vi "LVDimInterface.dim_set_DNS_node.vi"(1 "DNS node":string, 5 "error in (no error)":errorcluster) -> (14 "success":i32, 19 "error out":errorcluster)   [LabVIEW 2014, in "LVDimInterface.lvlib"]
doc: "This routine can be called by a server or a client program before publishing or subscribing to any services in order to programmatically declare the node where the DNS is running. If this call is not used the environment variable DIM_DNS_NODE will be used instead.\n\nA list of node names separated by commas can be given as a parameter, in which case the server or the client will use the first name server found running from the list.\n\n\n\nHistory: 29-JUN-2006, Dietrich Beck\n\nCopyright (C)\nGesellschaft für Schwerionenforschung, GSI\nPlanckstr. 1\n64291 Darmstadt\nGermany\n\nContact: D.Beck@gsi.de \n\nThis program is free software; you can redistribute it and/or modify it under the terms of the \nGNU General Public License as published by the Free Software Foundation; either version 2 of the license, or (at your option) any later version.\n\nThis program is distributed in the hope that it will be useful, but WITHOUT ANY WARRANTY; without even the implied warranty of MERCHANTABILITY or FITNESS FOR A PARTICULAR PURPOSE. See the GNU General License for more details (http://www.gnu.org).\n\nGesellschaft für Schwerionenforschung, GSI\nPlanckstr. 1, 64291 Darmstadt, Germany\nFor all questions and ideas contact D. Beck.\nLast update: 16-DEC-2005"
uses:
  LVDimInterface.lvlib
  bin/libDimWrapper.dll
  bin/libDimWrapper.so
  bin/libDimWrapperSPL.dll
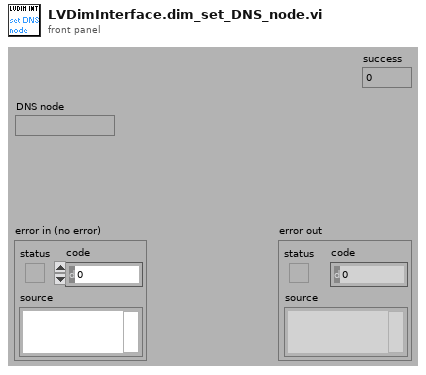
[diagram p1: front panel]
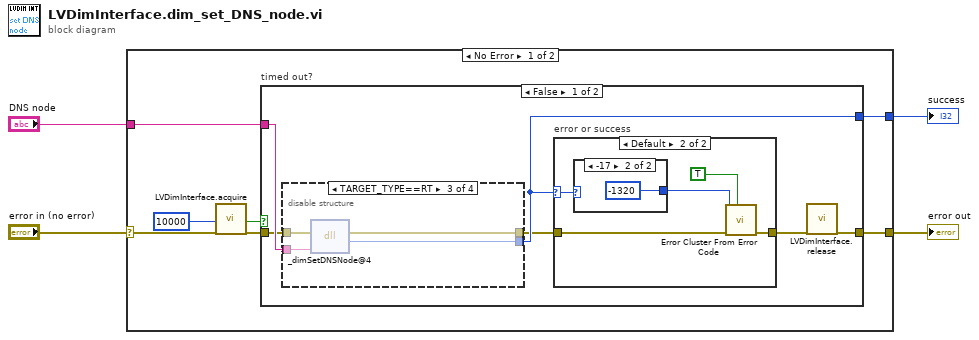
[diagram p0: block diagram]
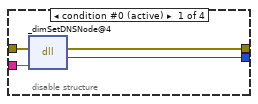
[diagram p2: hidden frame]
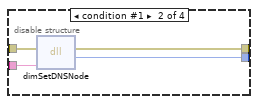
[diagram p3: hidden frame]
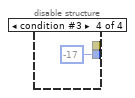
[diagram p4: hidden frame]
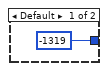
[diagram p6: hidden frame]
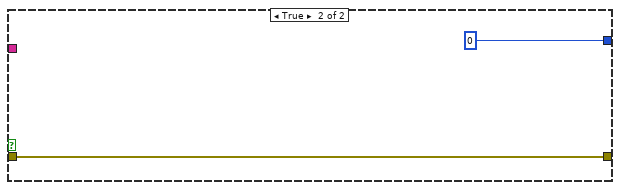
[diagram p7: hidden frame]
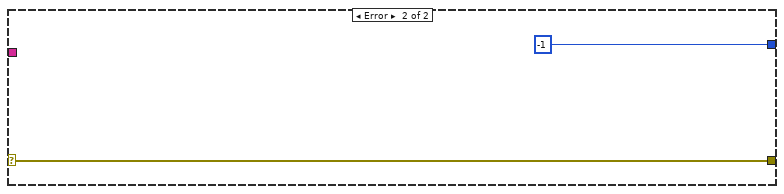
[diagram p8: hidden frame]
diagram:
  n1 = case shown="No Error" "error in (no error)" {
    selector: "error in (no error)" -> [w5 w42]
    tunnel: "DNS node" -> [w11 _]
    tunnel: [w10 -1 ("success")] -> w3
    tunnel: [w9 w42] -> w2
    frame No Error {
      n2 = call "LVDimInterface.acquire.vi"("ms timeout (10000)"=10000 ("ms timeout (-1)"), "error in (no error)"=w5) -> ("timed out"=w7:bool, "error out"=w8:errorcluster)  [unwired: 16 in]
      n3 = case "timed out?" shown="False" w7 {
        tunnel: w11 -> [w17 _]
        tunnel: [w16 0 ("success")] -> w10
        tunnel: [w12 w39] -> w9
        tunnel: w8 -> [w14 w39]
        frame False {
          n4 = disable-structure "Conditional Disable Structure" shown="TARGET_TYPE==RT" {
            disable-tunnel: w17 -> [w21 w25 w29 _]
            disable-tunnel: [w20 w24 w28 -17 ("success")] -> w16
            disable-tunnel: w14 -> [w19 w23 w27 _]
            disable-tunnel: [w18 w22 w26 _] -> w15
            frame condition #0 (active) {
              n5 = dll-call lib="D:/Git/CS-framework/CSlibraries/DimLVEvent/bin/libDimWrapper.dll" fn="_dimSetDNSNode@4" label="dimSetDNSNode"(error in=w19, "DNSNode"=w21) -> (error out=w18:errorcluster, "success"=w20:i32)  [unwired: 3 in, 1 out]
            }
            frame condition #1 {
              n6 = dll-call lib="D:/Git/CS-framework/CSlibraries/DimLVEvent/bin/libDimWrapper.so" fn="dimSetDNSNode"(error in=w23, "DNSNode"=w25) -> (error out=w22:errorcluster, "success"=w24:i32)  [unwired: 3 in, 1 out]
            }
            frame condition #2 {
              n7 = dll-call lib="D:/Git/CS-framework/CSlibraries/DimLVEvent/bin/libDimWrapperSPL.dll" fn="_dimSetDNSNode@4" label="libDimWrapper.so:dimSetDNSNode"(error in=w27, "DNSNode"=w29) -> (error out=w26:errorcluster, "success"=w28:i32)  [unwired: 3 in, 1 out]
            }
            frame condition #3 {
            }
          }
          n8 = case "error or success" shown="Default" w16 {
            selector: w16 -> [_ w36]
            tunnel: w15 -> [w31 w35]
            tunnel: [w31 w34] -> w13
            frame 1 {
            }
            frame Default {
              n9 = case shown="-17" w36 {
                tunnel: [-1319 ("code") -1320 ("code")] -> w32
                frame Default {
                }
                frame -17 {
                }
              }
              n10 = call <vilib>:"Error Cluster From Error Code.vi"("show call chain? (False)"=TRUE ("status"), "error in (no error)"=w35, "error code (0)"=w32) -> ("error out"=w34:errorcluster)  [unwired: 6 in]
            }
          }
          n11 = call "LVDimInterface.release.vi"("error in (no error)"=w13) -> ("error out"=w12:errorcluster)  [unwired: 18 in]
        }
        frame True {
        }
      }
    }
    frame Error {
    }
  }
  "error out" <- w2
  "success" <- w3
